vi "FPGA_I2C_Read.vi"(6 "Bytes To Read":u16=8, 8 "error in":errorcluster, 9 "I2C_Address":u16, 10 "Port":u8, 11 "FPGA VI Reference":T1) -> (0 "error out":errorcluster, 2 "Read Data":u8[](array[numeric]), 3 "FPGA VI Reference Out":T1)   [LabVIEW 2020, in "I2C Host API.lvlib"]
doc: "Returns <b>Bytes to Read</b> number of bytes, most significant bit first from the specified port and address."
uses:
  I2C Host API.lvlib
  RT/Controls/FPGA I2C_FPGA Ref.ctl
  FPGA/Controls/FPGA I2C_Cmd.ctl
  <vilib>/Utility/error.llb/Error Cluster From Error Code.vi
  <vilib>/rvi/errors/niLvFpgaAdjustHostInterfaceError.vi
  <vilib>/rvi/interface/nirviReadWriteControl/nirviReadWriteControl.xnode
  FPGA Bitfiles/I2CCommunication_FPGATarget2_I2CCommunication_VvdNkCkGvgg.lvbitx
  FPGA/FPGA-Main.vi
  NiFpgaLv.dll
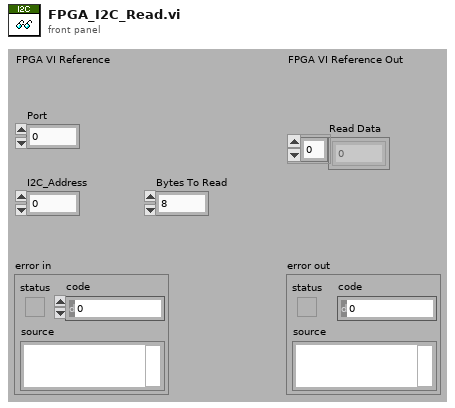
[diagram p1: front panel]
types:
  T1 = typedef "FPGA I2C_FPGA Ref.ctl" = refnum<k20>
  T2 = typedef "FPGA I2C_Cmd.ctl" = enum8{"Idle", "Write I2C", "Read I2C", "Write & Read I2C", "Configure"}
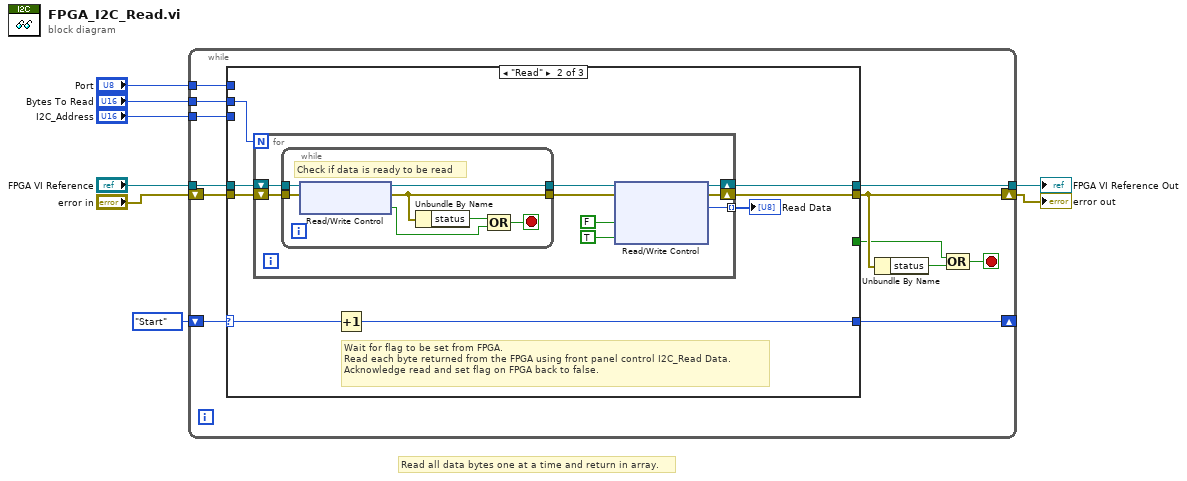
[diagram p0: block diagram]
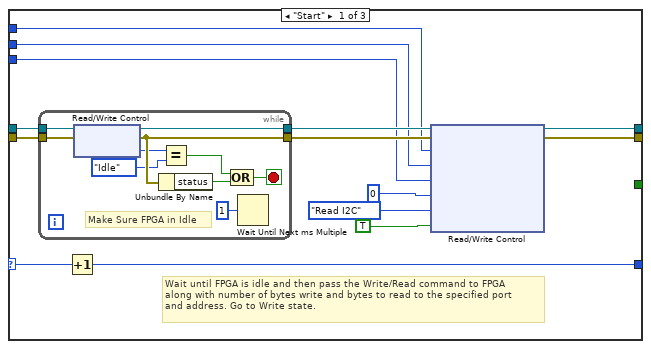
[diagram p2: hidden frame]
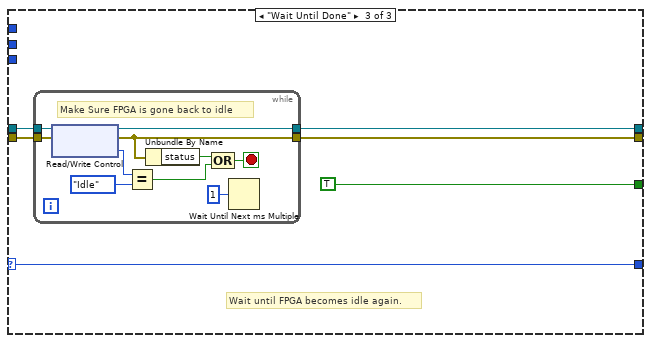
[diagram p3: hidden frame]
diagram:
  # "Read all data bytes one at a time and return in array."
  n1 = while {
    tunnel: "FPGA VI Reference" -> [w20]
    tunnel: [w18] -> w7
    shift-right: [w17] -> w6
    shift-left: "error in" -> [w19]
    shift-right: [w12] -> _
    shift-left: enum16{"Start", "Read", "Wait Until Done"}."Start" -> [w13]
    tunnel: "Bytes To Read" -> [w11]
    tunnel: "Port" -> [w10]
    tunnel: "I2C_Address" -> [w9]
    stop <- w14 stop-if-true
    n2 = case shown="\"Read\"" w13 {
      selector: w13 -> [w28 w47 w70]
      tunnel: w20 -> [w32 w51 w74]
      tunnel: w19 -> [w31 w50 w73]
      tunnel: [w29 w49 w72] -> w18
      tunnel: [w30 w48 w71] -> w17
      tunnel: [_ _ TRUE] -> w16
      tunnel: [w27 w46 w70] -> w12
      tunnel: w11 -> [w26 w45 _]
      tunnel: w10 -> [w25 _ _]
      tunnel: w9 -> [w24 _ _]
      frame "Start" {
        # "Wait until FPGA is idle and then pass the Write/Read command to FPGA\nalong with number of bytes write and bytes to read to the specified port\nand address. Go to Write state."
        n3 = while {
          tunnel: w32 -> [w44]
          tunnel: [w43] -> w34
          tunnel: w31 -> [w42]
          tunnel: [w39] -> w33
          stop <- w40 stop-if-true
          # "Make Sure FPGA in Idle"
          n4 = xnode "Read/Write Control"("FPGA VI Reference In"=w44, "error in"=w42) -> ("FPGA VI Reference Out"=w43:T1, "error out"=w39:errorcluster, "I2C_Cmd"=w37:T2)
          n5 = Unbundle By Name(w39) -> ("status"=w41:bool)
          n6 = Equal?(x=w37, y=FPGA_I2C_Cmd."Idle" ("I2C_Cmd")) -> (x = y?=w38:bool)
          n7 = Compound Arithmetic op=OR(w38, w41) -> (w40:bool)
          n8 = Wait Until Next ms Multiple(millisecond multiple=u32 1) -> ()  [unwired: 1 out]
        }
        n9 = Increment(x=w28) -> (x+1=w27:enum16{"Start", "Read", "Wait Until Done"})
        n10 = xnode "Read/Write Control"("FPGA VI Reference In"=w34, "error in"=w33, "I2C_Port"=w25, "I2C_Bytes to Read"=w26, "I2C_Address"=w24, "I2C_Bytes to Write"=u16 0, "I2C_Cmd"=FPGA_I2C_Cmd."Read I2C", "I2C_Start"=TRUE ("Start")) -> ("FPGA VI Reference Out"=w29:T1, "error out"=w30:errorcluster)
      }
      frame "Read" {
        # "Wait for flag to be set from FPGA.\nRead each byte returned from the FPGA using front panel control I2C_Read Data.\nAcknowledge read and set flag on FPGA back to false."
        n11 = for {
          N: w45 -> [_]
          shift-right: [w57] -> w49
          shift-left: w51 -> [w61]
          shift-right: [w56] -> w48
          shift-left: w50 -> [w60]
          tunnel: [w55] -> w52 mode=indexing
          n12 = while {
            tunnel: w61 -> [w63]
            tunnel: w60 -> [w68]
            tunnel: [w67] -> w59
            tunnel: [w66] -> w58
            stop <- w64 stop-if-true
            # "Check if data is ready to be read"
            n13 = xnode "Read/Write Control"("FPGA VI Reference In"=w63, "error in"=w68) -> ("FPGA VI Reference Out"=w67:T1, "error out"=w66:errorcluster, "I2C_Read Flag"=w62:bool)
            n14 = Unbundle By Name(w66) -> ("status"=w65:bool)
            n15 = Compound Arithmetic op=OR(w65, w62) -> (w64:bool)
          }
          n16 = xnode "Read/Write Control"("FPGA VI Reference In"=w59, "error in"=w58, "I2C_Read Flag"=FALSE ("Read Flag"), "I2C_Ack Read"=TRUE ("Write Flag")) -> ("FPGA VI Reference Out"=w57:T1, "error out"=w56:errorcluster, "I2C_Read Data"=w55:u8)
        }
        "Read Data" <- w52
        n17 = Increment(x=w47) -> (x+1=w46:enum16{"Start", "Read", "Wait Until Done"})
      }
      frame "Wait Until Done" {
        # "Wait until FPGA becomes idle again."
        n18 = while {
          tunnel: w74 -> [w84]
          tunnel: [w83] -> w72
          tunnel: w73 -> [w82]
          tunnel: [w80] -> w71
          stop <- w77 stop-if-true
          # "Make Sure FPGA is gone back to idle"
          n19 = xnode "Read/Write Control"("FPGA VI Reference In"=w84, "error in"=w82) -> ("FPGA VI Reference Out"=w83:T1, "error out"=w80:errorcluster, "I2C_Cmd"=w81:T2)
          n20 = Equal?(x=w81, y=FPGA_I2C_Cmd."Idle") -> (x = y?=w78:bool)
          n21 = Unbundle By Name(w80) -> ("status"=w79:bool)
          n22 = Compound Arithmetic op=OR(w79, w78) -> (w77:bool)
          n23 = Wait Until Next ms Multiple(millisecond multiple=u32 1) -> ()  [unwired: 1 out]
        }
      }
    }
    n24 = Unbundle By Name(w17) -> ("status"=w15:bool)
    n25 = Compound Arithmetic op=OR(w16, w15) -> (w14:bool)
  }
  "FPGA VI Reference Out" <- w7
  "error out" <- w6
